vi "test Verify No Timestamp Channels.vi"(8 "error in":errorcluster, 11 "TestCase in":refnum<class "Scripting.lvclass">=refnum) -> (0 "error out":errorcluster, 3 "TestCase out":refnum<class "Scripting.lvclass">)   [LabVIEW 2020, in "Scripting.lvclass"]
uses:
  Scripting.lvclass
  <vilib>/addons/_JKI Toolkits/VI Tester/TestCase.llb/TestCase.lvclass
  Scripting/AIM MIL-STD-1553 Scripting.lvlib
  Shared/Address.ctl
  Shared/Message Type.ctl
  Shared/Terminal Endpoint.ctl
  Shared/Parameter Definition.ctl
  Shared/Message Definition.ctl
  Shared/1553 Channel.ctl
  Scripting/Constants.vi
  <vilib>/NI VeriStand/Custom Device Tools/Custom Device Utility Library/Custom Device Utility Library.lvlib
  <vilib>/NI VeriStand/Custom Device Tools/Custom Device Utility Library/NI VeriStand - Search for All Items by GUID.vi
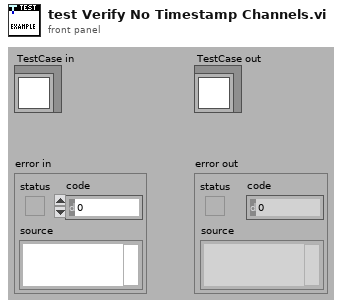
[diagram p1: front panel]
types:
  T1 = typedef "1553 Channel.ctl" = cluster{"HW channel":u16, "terminal addresses":T2[], "terminal names":string[], "acyclic frame names":string[], "messages":T3[]}
  T2 = typedef "Address.ctl" = u16
  T3 = typedef "Message Definition.ctl" = cluster{"name":string, "message type":T4, "endpoint Tx":T5, "endpoint Rx":T5, "create timestamp channel":bool, "mode code":u16, "number of words":u16, "parameters":cluster{"name":string, "default value":dbl, "unit":string, "parameter definition":T6}[]}
  T4 = typedef "Message Type.ctl" = string
  T5 = typedef "Terminal Endpoint.ctl" = cluster{"terminal address":T2, "subaddress":T2}
  T6 = typedef "Parameter Definition.ctl" = cluster{"start index":i32, "size (bits)":i32, "encoding":enum16{"BNR", "BCD", "Discrete"}, "signed":bool, "multiplier":dbl, "offset":dbl}
  T7 = typedef "Custom Device API.lvlib/Custom Device Item Ref.ctl" = u64
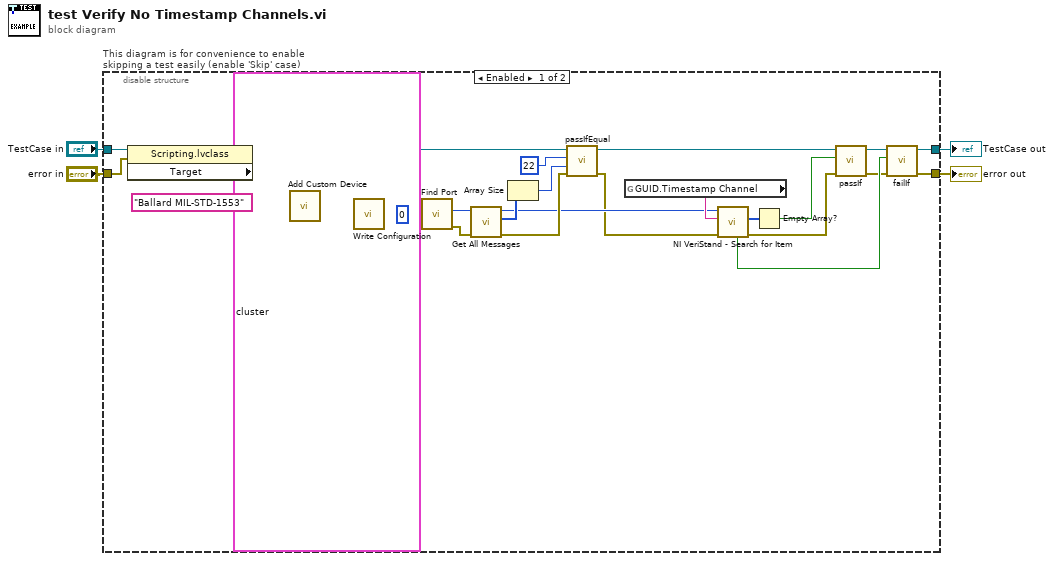
[diagram p0: block diagram]
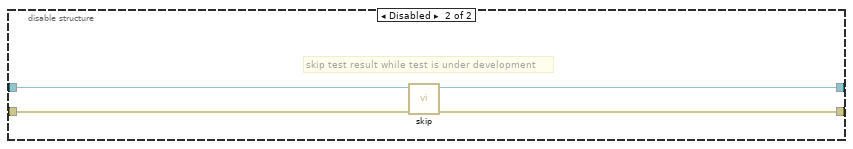
[diagram p2: hidden frame]
diagram:
  n1 = disable-structure "This diagram is for convenience to enable skipping a test easily (enable 'Skip' case)" shown="Enabled" {
    disable-tunnel: "TestCase in" -> [w33 w38]
    disable-tunnel: [w5 w36] -> w1
    disable-tunnel: [w6 w37] -> w3
    disable-tunnel: "error in" -> [w28 w35]
    frame Enabled {
      n2 = property class="Scripting.lvclass"(reference=w33, error in=w28) -> (reference out=w19:refnum<class "Scripting.lvclass">, error out=w27:errorcluster, "Target"=w32)
      n3 = call "Add Custom Device.vi"("error in"=w27, "name"="Ballard MIL-STD-1553", "target in"=w32) -> ("error out"=w29:errorcluster, "Ballard MIL-STD 1553 custom device"=w31:T7)  [unwired: 6 in, 1 out]
      n4 = call "Write Configuration.vi"("error in"=w29, "1553 channels"=T1[] [{"HW channel"=0, "terminal addresses"=[0, 1, 15, 21, 31], "terminal names"=[], "acyclic frame names"=["acyclicFrame ID56"], "messages"=[{"name"="BC to RT 1.2", "message type"="BC to RT", "endpoint Tx"={"terminal address"=0, "subaddress"=0}, "endpoint Rx"={"terminal address"=1, "subaddress"=2}, "create timestamp channel"=FALSE, "mode code"=0, "number of words"=3, "parameters"=[]}, {"name"="RT 31.15 to RT 21.21", "message type"="RT to RT", "endpoint Tx"={"terminal address"=15, "subaddress"=21}, "endpoint Rx"={"terminal address"=31, "subaddress"=21}, "create timestamp channel"=FALSE, "mode code"=0, "number of words"=11, "parameters"=[]}, {"name"="BC to RT 1.3", "message type"="BC to RT", "endpoint Tx"={"terminal address"=0, "subaddress"=0}, "endpoint Rx"={"terminal address"=1, "subaddress"=3}, "create timestamp channel"=FALSE, "mode code"=0, "number of words"=4, "parameters"=[]}, {"name"="RT 1.5 to BC", "message type"="RT to BC", "endpoint Tx"={"terminal address"=1, "subaddress"=5}, "endpoint Rx"={"terminal address"=0, "subaddress"=0}, "create timestamp channel"=FALSE, "mode code"=0, "number of words"=6, "parameters"=[]}, {"name"="RT 1.6 to BC", "message type"="RT to BC", "endpoint Tx"={"terminal address"=1, "subaddress"=6}, "endpoint Rx"={"terminal address"=0, "subaddress"=0}, "create timestamp channel"=FALSE, "mode code"=0, "number of words"=2, "parameters"=[]}, {"name"="RT 1.20 to RT 15.20", "message type"="RT to RT", "endpoint Tx"={"terminal address"=1, "subaddress"=20}, "endpoint Rx"={"terminal address"=15, "subaddress"=20}, "create timestamp channel"=FALSE, "mode code"=0, "number of words"=4, "parameters"=[]}, {"name"="MC 16", "message type"="MC", "endpoint Tx"={"terminal address"=1, "subaddress"=31}, "endpoint Rx"={"terminal address"=0, "subaddress"=0}, "create timestamp channel"=FALSE, "mode code"=16, "number of words"=1, "parameters"=[]}, {"name"="MC 17", "message type"="MC", "endpoint Tx"={"terminal address"=0, "subaddress"=0}, "endpoint Rx"={"terminal address"=1, "subaddress"=31}, "create timestamp channel"=FALSE, "mode code"=17, "number of words"=1, "parameters"=[]}, {"name"="BC to RT 31.28", "message type"="BC to RT", "endpoint Tx"={"terminal address"=0, "subaddress"=0}, "endpoint Rx"={"terminal address"=31, "subaddress"=28}, "create timestamp channel"=FALSE, "mode code"=0, "number of words"=6, "parameters"=[]}, {"name"="MC 1", "message type"="MC", "endpoint Tx"={"terminal address"=0, "subaddress"=0}, "endpoint Rx"={"terminal address"=31, "subaddress"=31}, "create timestamp channel"=FALSE, "mode code"=1, "number of words"=0, "parameters"=[]}]}], "Ballard MIL-STD 1553 custom device in"=w31) -> ("error out"=w22:errorcluster, "Ballard MIL-STD 1553 custom device out"=w24:T7)  [unwired: 7 in]
      n5 = call "Find Port.vi"("error in"=w22, "port number"=u16 0, "Ballard MIL-STD 1553 custom device in"=w24) -> ("error out"=w17:errorcluster, "port"=w18:T7)  [unwired: 5 in, 2 out]
      n6 = call "Get All Messages.vi"("error in"=w17, "port in"=w18) -> ("error out"=w20:errorcluster, "messages"=w21:T7[], "port out"=w15:T7)  [unwired: 7 in]
      n7 = Array Size(array=w21) -> (size(s)=w26:i32)
      n8 = call-dynamic "passIfEqual.vi"("error in (no error)"=w20, "y"=w26, "x"=22 ("size(s)"), "TestCase in"=w19) -> ("error out"=w14:errorcluster, "TestCase out"=w13:refnum<class "Scripting.lvclass">)  [unwired: 6 in]
      n9 = global read "Constants.vi" "GUID.Timestamp Channel"() -> (w16:string)
      n10 = call-poly <vilib>:"NI VeriStand - Search for Item.vi"("error in"=w14, "Item GUID"=w16, "Section Ref in"=w15) -> ("error out"=w12:errorcluster, "Item Refs"=w11:T7[], "Found"=w9:bool)  [unwired: 5 in, 1 out]
      n11 = Empty Array?(array=w11) -> (empty?=w10:bool)
      n12 = call-dynamic "passIf.vi"("error in (no error)"=w12, "pass"=w10, "TestCase in"=w13) -> ("error out"=w7:errorcluster, "TestCase out"=w8:refnum<class "Scripting.lvclass">)  [unwired: 7 in]
      n13 = call-dynamic "failIf.vi"("error in (no error)"=w7, "fail"=w9, "TestCase in"=w8) -> ("error out"=w6:errorcluster, "TestCase out"=w5:refnum<class "Scripting.lvclass">)  [unwired: 7 in]
    }
    frame Disabled {
      # "skip test result while test is under development"
      n14 = call <vilib>:"skip.vi"("error in (no error)"=w35, "TestCase in"=w38) -> ("error out"=w37:errorcluster, "TestCase out"=w36:refnum<class "TestCase.lvclass">)  [unwired: 8 in]
    }
  }
  "error out" <- w3
  "TestCase out" <- w1
